vi "CTL 5PtCalControl.vi"(7 "Full Cfg 2":T2, 8 "Cal State In":T1, 9 "Laser Raw":dbl=26.450000000001474, 10 "Level SP":dbl=8.0, 11 "Level PV":dbl=26.450000000001474) -> (0 "Cal State Out":T1)   [LabVIEW 2024]
doc: "Simulates the level inch (0 = empty) and Level Sense (8.5 = empty).\nIf Test Status is manual then the Drain and Fill buttons cause the level to decrese or increase.\nOtherwise, drain and fill are determnied by the state variable and the difference between Level SP (Set Point) and Level PV (Present Value)\nThe level rate of change is determined by the Flow Rate setting."
uses:
  Control Definitions/Def FullCfg.ctl
  Control Definitions/Def BenchCfg.ctl
  Control Definitions/Def PumpCtlRefs.ctl
  Control Definitions/Def_PumpSpeed.ctl
  Control Definitions/Def Bench Status.ctl
  Control Definitions/DEF_5ptCalState.ctl
panel:
  out "error out":errorcluster
  in  "error in (no error)":errorcluster
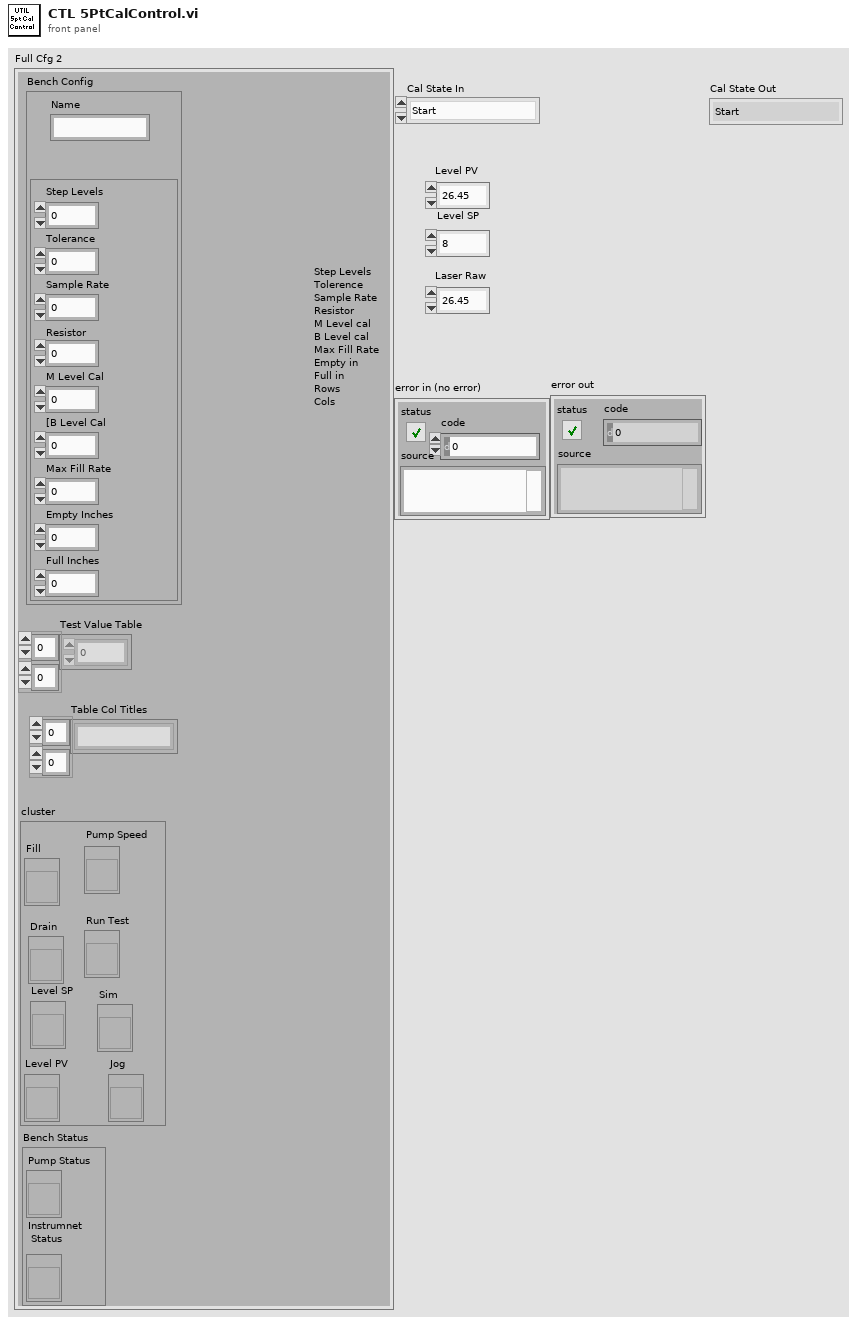
[diagram p1: front panel]
types:
  T1 = typedef "DEF_5ptCalState.ctl" = enum16{"Start", "Load Tester", "Go Auto", "Level 1", "Reveiw ", "Save", "Exit"}
  T2 = typedef "Def FullCfg.ctl" = cluster{"Bench Config":T3, "Test Value Table ":dbl[][], "Table Col Titles":string[][], "cluster":T4, "Bench Status":T5}
  T3 = typedef "Def BenchCfg.ctl" = cluster{"Name":string, cluster{"Step Levels":dbl, "Tolerance":dbl, "Sample Rate":dbl, "Resistor":dbl, "M Level Cal":dbl, "[B Level Cal":dbl, "Max Fill Rate":dbl, "Empty Inches":dbl, "Full Inches":dbl}}
  T4 = typedef "Def PumpCtlRefs.ctl" = cluster{"Fill ":refnum<vi>, "Drain":refnum<vi>, "Level PV":refnum<vi>, "Pump Speed":refnum<vi>, "Run Test":refnum<vi>, "Sim":refnum<vi>, "Jog":refnum<vi>, "Level SP":refnum<vi>}
  T5 = typedef "Def Bench Status.ctl" = cluster{"Pump Status":refnum<vi>, "Instrumnet\n Status":refnum<vi>}
  T6 = cluster{"Step Levels":dbl, "Tolerance":dbl, "Sample Rate":dbl, "Resistor":dbl, "M Level Cal":dbl, "[B Level Cal":dbl, "Max Fill Rate":dbl, "Empty Inches":dbl, "Full Inches":dbl}
  T7 = cluster{"Level SP":dbl, "Level PV":dbl, "Full Inches":dbl, "Empty Inches":dbl, "Laser Raw":dbl}
  T8 = typedef "Def_PumpCmds.ctl" = cluster{"Set Point":dbl, "Drain":bool, "Fill":bool, "Pump Speed ":T9}
  T9 = typedef "Def_PumpSpeed.ctl" = enum16{"FAST", "SLOW", "CREEP", "STOP"}
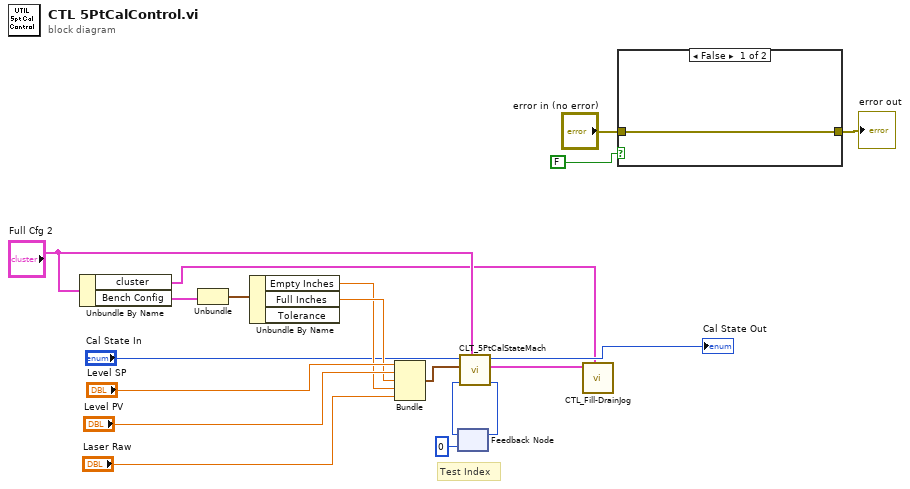
[diagram p0: block diagram]
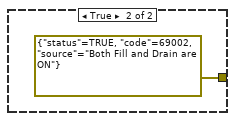
[diagram p2: hidden frame]
diagram:
  # "Test Index"
  n1 = Unbundle By Name("Full Cfg 2") -> ("cluster"=w3:T4, "Bench Config"=w17:T3)
  n2 = Unbundle(w17) -> (w16:T6)  [unwired: 1 out]
  n3 = Unbundle By Name(w16) -> ("Empty Inches"=w12:dbl, "Full Inches"=w13:dbl)  [unwired: 1 out]
  n4 = Bundle("Level SP"="Level SP", "Level PV"="Level PV", "Full Inches"=w13, "Empty Inches"=w12, "Laser Raw"="Laser Raw") -> (w11:T7)  [unwired: 1 in]
  n5 = feedback #1(0 ("Index Out")) -> (w2:i32)
  n6 = call "CLT_5PtCalStateMach.vi"("Full Cfg"="Full Cfg 2", "Index In"=w2, "Pump Signals"=w11, "Cal State In"="Cal State In") -> ("Index Out"=w1:i32, "Pump Cmds"=w8:T8, "Cal State Out"=→"Cal State Out":T1)  [unwired: 5 in]
  n7 = feedback-in #1(w1) -> ()
  n8 = call "CTL_Fill-DrainJog.vi"("Pump CtlRef In"=w3, "Pump Cmds"=w8) -> ()  [unwired: 6 in, 4 out]
  n9 = case shown="False" FALSE {
    tunnel: "error in (no error)" -> [w20 _]
    tunnel: [w20 errorcluster {"status"=TRUE, "code"=69002, "source"="Both Fill and Drain are ON"} ("error in (no error)")] -> w18
    frame False {
    }
    frame True {
    }
  }
  "error out" <- w18
